vi "输入信息.vi"(8 "error in (no error)":errorcluster caption="错误输入（无错误）", 11 "输入信息":string) -> (0 "error out":errorcluster caption="错误输出")   [LabVIEW 2011, in "单例.lvlib"]
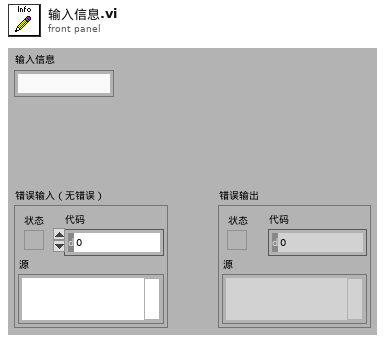
[diagram p1: front panel]
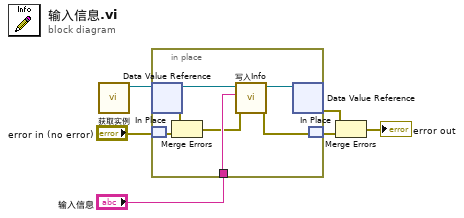
[diagram p0: block diagram]
diagram:
  n1 = call "获取实例.vi"() -> ("data value reference"=w6:refnum<data-value>)  [unwired: 11 in]
  n2 = in-place {
    in-place-border: "输入信息" -> [w11]
    n3 = in-place-dvr #1(w6) -> (w13:refnum<class "单例.lvclass">, w10:errorcluster)
    n4 = in-place-match #2("error in (no error)") -> (w9:errorcluster)
    n5 = Merge Errors(w10, w9) -> (w8:errorcluster)
    n6 = call "写入Info.vi"("error in (no error)"=w8, "Info"=w11, "单例输入"=w13) -> ("error out"=w7:errorcluster, "单例输出"=w12:refnum<class "单例.lvclass">)  [unwired: 7 in]
    n7 = in-place-dvr #1(w12) -> (w2:errorcluster)  [unwired: 1 out]
    n8 = in-place-match #2(w7) -> (w3:errorcluster)
  }
  n9 = Merge Errors(w2, w3) -> (→"error out":errorcluster)
